vi "convertps--mm-minusSD.vi"(1 "mm":dbl) -> (0 "ps":dbl)   [LabVIEW 2015]
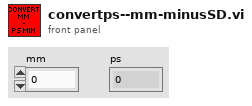
[diagram p1: front panel]
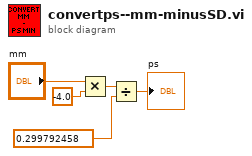
[diagram p0: block diagram]
diagram:
  n1 = Multiply(x="mm", y=-4.0) -> (x*y=w1:dbl)
  n2 = Divide(x=w1, y=0.299792458) -> (x/y=→"ps":dbl)
